vi "create GWS srm config.vi"(4 "error in (no error)":errorcluster) -> (0 "error out":errorcluster)   [LabVIEW 2011]
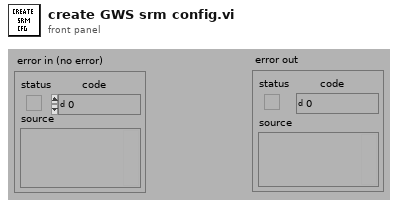
[diagram p1: front panel]
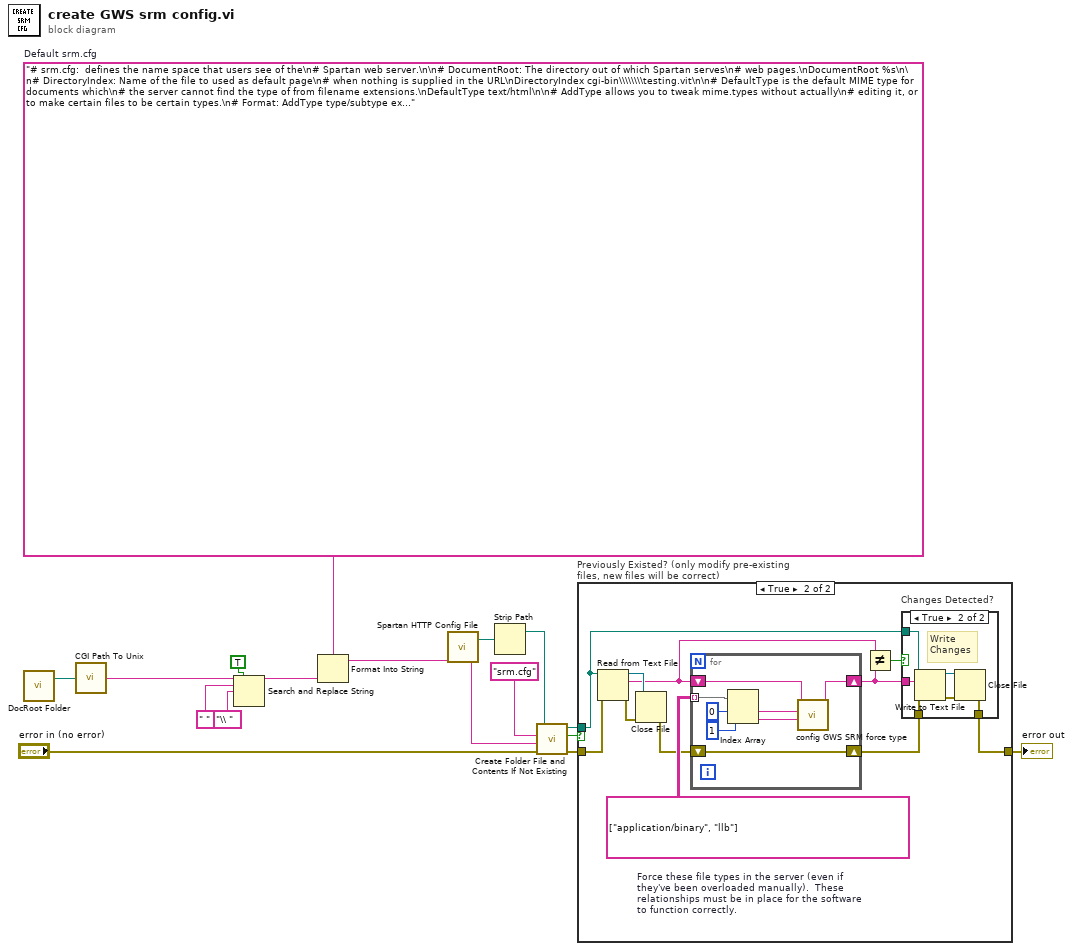
[diagram p0: block diagram]
diagram:
  w5 = "# srm.cfg:  defines the name space that users see of the\n# Spartan web server.\n\n# DocumentRoot: The directory out of which Spartan serves\n# web pages.\nDocumentRoot %s\n\n# DirectoryIndex: Name of the file to used as default page\n# when nothing is supplied in the URL\nDirectoryIndex cgi-bin\\\\\\\\testing.vit\n\n# DefaultType is the default MIME type for documents which\n# the server cannot find the type of from filename extensions.\nDefaultType text/html\n\n# AddType allows you to tweak mime.types without actually\n# editing it, or to make certain files to be certain types.\n# Format: AddType type/subtype ext1\n\n# Cascading stylesheets\nAddType text/css css\n\n# Enable VIs as CGIs support\nAddType application/x-lvhttp-cgi vi\n\n# Enable binary executable (.exe) and\n# dynamic library (.dll) and\n# pdf document (.pdf) downloads\nAddType application/octet-stream exe\nAddType application/binary dll\nAddType application/binary llb\nAddType application/pdf pdf\n\n# Enable builtin image map support\nAddType text/x-imagemap map\n\n\n# Enable HTML Components\nAddType text/x-component htc\n\n# Enable XML Components\nAddType text/xml xml\n\n# AddEncoding allows you to have certain browsers (Mosaic/X 2.1+) uncompress\n# information on the fly. Note: Not all browsers support this.\nAddEncoding x-compress Z\nAddEncoding x-gzip gz\n"  # Default srm.cfg
  n1 = call "DocRoot Folder.vi"() -> ("DocumentRoot Folder"=w2:path)  [unwired: 3 in]
  n2 = call "CGI Path To Unix.vi"("platform path"=w2) -> ("unix path"=w6:string)  [unwired: 1 in]
  n3 = Search and Replace String(replace all?=TRUE ("replace all? (F)"), input string=w6, search string=" ", replace string="\\ " ("replace string (\"\")")) -> (result string=w3:string)  [unwired: 1 in, 6 out]
  n4 = Format Into String(format string=w5, w3) -> (resulting string=w4:string)  [unwired: 2 in, 1 out]
  n5 = call "Spartan HTTP Config File.vi"() -> ("HTTP Configuration File"=w14:path)  [unwired: 1 out]
  n6 = Strip Path(path=w14) -> (stripped path=w1:path)  [unwired: 1 out]
  n7 = call "Create Folder File and Contents If Not Existing.vi"("error in (no error)"="error in (no error)", "File contents to write (\"\")"=w4, "Filename (\"\")"="srm.cfg", "File Folder (Empty)"=w1) -> ("error out"=w13:errorcluster, "Already Existed?"=w10:bool, "Path to File"=w11:path)  [unwired: 1 out]
  n8 = case "Previously Existed? (only modify pre-existing files, new files will be correct)" shown="True" w10 {
    tunnel: w13 -> [w17 w27]
    tunnel: [w17 w25] -> w12
    tunnel: w11 -> [_ w18]
    frame False {
    }
    frame True {
      w28 = string[][] [["application/binary", "llb"]]  # Force these file types in the server (even if they've been overloaded manually).  These relationships must be in place for the software to function correctly.
      n9 = Read from Text File(file (use dialog)=w18, error in=w27) -> (refnum out=w24:refnum<file>, text=w21:string, error out=w23:errorcluster)  [unwired: 2 in, 1 out]
      n10 = Close File(refnum=w24, error in=w23) -> (error out=w22:errorcluster)  [unwired: 1 out]
      n11 = for {
        shift-right: [w43] -> w26
        shift-left: w22 -> [w43]
        shift-right: [w36] -> w20
        shift-left: w21 -> [w37]
        tunnel: w28 -> [w42] mode=indexing
        n12 = Index Array(array=w42, index #1=0 ("index"), index #2=1 ("index")) -> (element #1=w39:string, element #2=w38:string)
        n13 = call "config GWS SRM force type.vi"("extension (w/o period)"=w38, "typeString (type/subtype)"=w39, "Configuration String In"=w37) -> ("Modified Configuration"=w36:string)  [unwired: 8 in]
      }
      n14 = Not Equal?(x=w21, y=w20) -> (x != y?=w19:bool)
      n15 = case "Changes Detected?" shown="True" w19 {
        tunnel: w26 -> [w29 w35]
        tunnel: [w29 w32] -> w25
        tunnel: w20 -> [_ w31]
        tunnel: w18 -> [_ w30]
        frame False {
          # "Do\nNothing"
        }
        frame True {
          # "Write\nChanges"
          n16 = Write to Text File(file (use dialog)=w30, text=w31, error in=w35) -> (refnum out=w33:refnum<file>, error out=w34:errorcluster)  [unwired: 1 in, 1 out]
          n17 = Close File(refnum=w33, error in=w34) -> (error out=w32:errorcluster)  [unwired: 1 out]
        }
      }
    }
  }
  "error out" <- w12
